vi "MCCPMTstore.vi"(0 "MCCPMT in":refnum<class "MCCPMT.lvclass">, 5 "pmt voltage 1":dbl, 7 "pmt voltage 2":dbl, 9 "pmt voltage 3":dbl, 11 "error in (no error)":errorcluster) -> (4 "MCCPMT out":refnum<class "MCCPMT.lvclass">, 15 "error out":errorcluster)   [LabVIEW 2012, in "MCCPMT.lvclass"]
uses:
  MCCPMT.lvclass
  MCCPMT.lvclass/MCCPMT.ctl
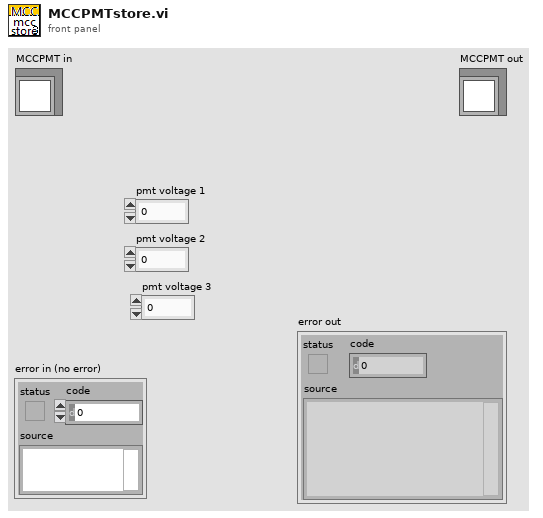
[diagram p1: front panel]
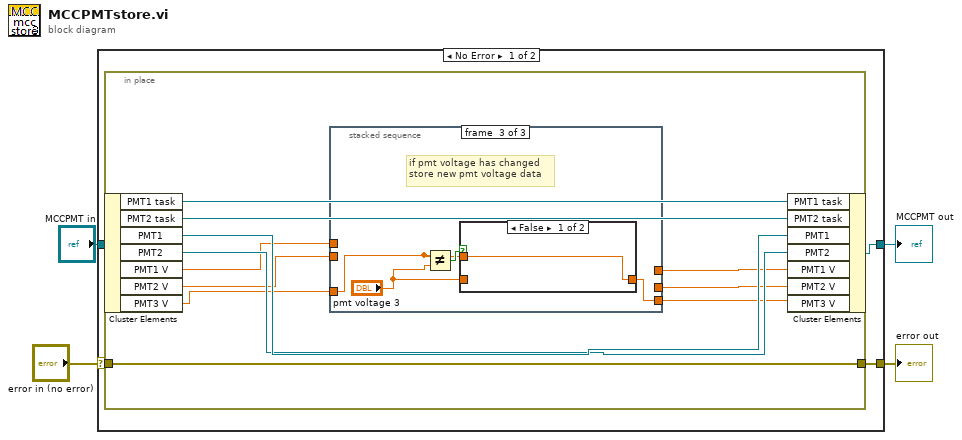
[diagram p0: block diagram]
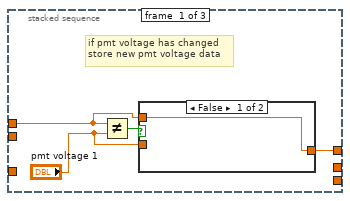
[diagram p2: hidden frame]
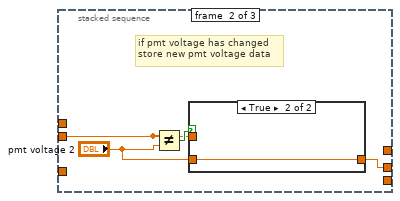
[diagram p4: hidden frame]
diagram:
  n1 = case shown="No Error" "error in (no error)" {
    selector: "error in (no error)" -> [w6 w39]
    tunnel: [w5 w39] -> w3
    tunnel: [w7 w38] -> w1
    tunnel: "MCCPMT in" -> [w8 w38]
    frame No Error {
      n2 = in-place {
        in-place-border: w6 -> [w19]
        in-place-border: [w19] -> w5
        n3 = in-place-cluster #1(w8) -> ("PMT1 task"=w16:refnum<k24>, "PMT2 task"=w15:refnum<k24>, "PMT1"=w18:refnum<k21>, "PMT2"=w17:refnum<k21>, "PMT1 V"=w14:dbl, "PMT2 V"=w12:dbl, "PMT3 V"=w9:dbl)
        n4 = stacked-sequence {
          tunnel: w14 -> [w20 _ _]
          tunnel: [w21 _ _] -> w13
          tunnel: w12 -> [_ w27 _]
          tunnel: [_ w26 _] -> w11
          tunnel: [_ _ w33] -> w10
          tunnel: w9 -> [_ _ w32]
          frame #0 {
            # "if pmt voltage has changed\nstore new pmt voltage data"
            n5 = Not Equal?(x=w20, y="pmt voltage 1") -> (x != y?=w23:bool)
            n6 = case shown="False" w23 {
              tunnel: "pmt voltage 1" -> [_ w25]
              tunnel: [w24 w25] -> w21
              tunnel: w20 -> [w24 _]
              frame False {
              }
              frame True {
              }
            }
          }
          frame #1 {
            # "if pmt voltage has changed\nstore new pmt voltage data"
            n7 = Not Equal?(x=w27, y="pmt voltage 2") -> (x != y?=w29:bool)
            n8 = case shown="True" w29 {
              tunnel: [w30 w31] -> w26
              tunnel: "pmt voltage 2" -> [_ w31]
              tunnel: w27 -> [w30 _]
              frame False {
              }
              frame True {
              }
            }
          }
          frame #2 {
            # "if pmt voltage has changed\nstore new pmt voltage data"
            n9 = Not Equal?(x=w32, y="pmt voltage 3") -> (x != y?=w35:bool)
            n10 = case shown="False" w35 {
              tunnel: [w36 w37] -> w33
              tunnel: "pmt voltage 3" -> [_ w37]
              tunnel: w32 -> [w36 _]
              frame False {
              }
              frame True {
              }
            }
          }
        }
        n11 = in-place-cluster #1("PMT1 task"=w16, "PMT2 task"=w15, "PMT1"=w18, "PMT2"=w17, "PMT1 V"=w13, "PMT2 V"=w11, "PMT3 V"=w10) -> (w7:refnum<class "MCCPMT.lvclass">)
      }
    }
    frame Error {
    }
  }
  "error out" <- w3
  "MCCPMT out" <- w1
